vi "arrayOfSoundsOrdered.vi"(11 "Array":string[](array[string])) -> (3 "name or relative path":string)   [LabVIEW 2019]
panel:
  in  "stop":bool
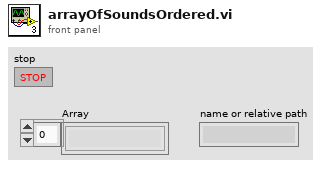
[diagram p1: front panel]
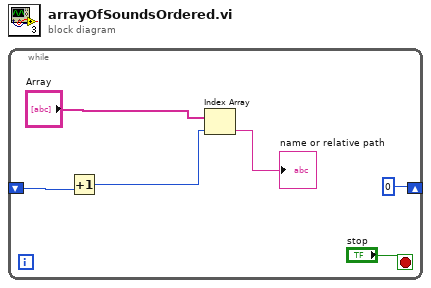
[diagram p0: block diagram]
diagram:
  n1 = while {
    shift-right: [0] -> _
    shift-left: _ -> [w3]
    stop <- "stop" stop-if-true
    n2 = Increment(x=w3) -> (x+1=w2:i32)
    n3 = Index Array(array="Array", index=w2) -> (element=→"name or relative path":string)
  }
